vi "Auton and Setpoints Selector.vi"() -> ()   [LabVIEW 2014]
uses:
  <vilib>/Rock Robotics/WPI/Joystick/WPI_JoystickGetSetRefNum.vi
  Robot Global Data.vi
  <vilib>/Rock Robotics/Network Tables/SD Write String.vi
  <vilib>/Rock Robotics/Network Tables/SD Write Number.vi
panel:
  out "Setpoints File Selected 2":string
  out "Auton File Selected":string
  out "Number of Auton Files":i64
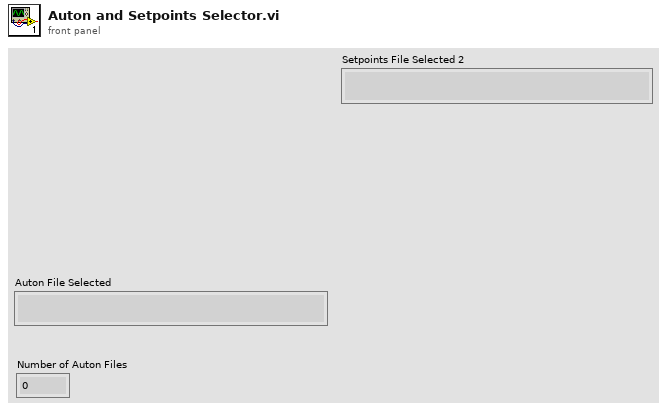
[diagram p1: front panel]
types:
  T1 = typedef "WPI_JoystickDevRef.ctl" = cluster{"Device":T2}
  T2 = typedef "WPI_JoystickDeviceEnum.ctl" = enum16{"USB 0", "USB 1", "USB 2", "USB 3", "USB 4", "USB 5"}
  T3 = cluster{"Buttons[0]":bool, "Buttons[1]":bool, "Buttons[2]":bool, "Buttons[3]":bool, "Buttons[4]":bool, "Buttons[5]":bool, "Buttons[6]":bool, "Buttons[7]":bool, "Buttons[8]":bool}
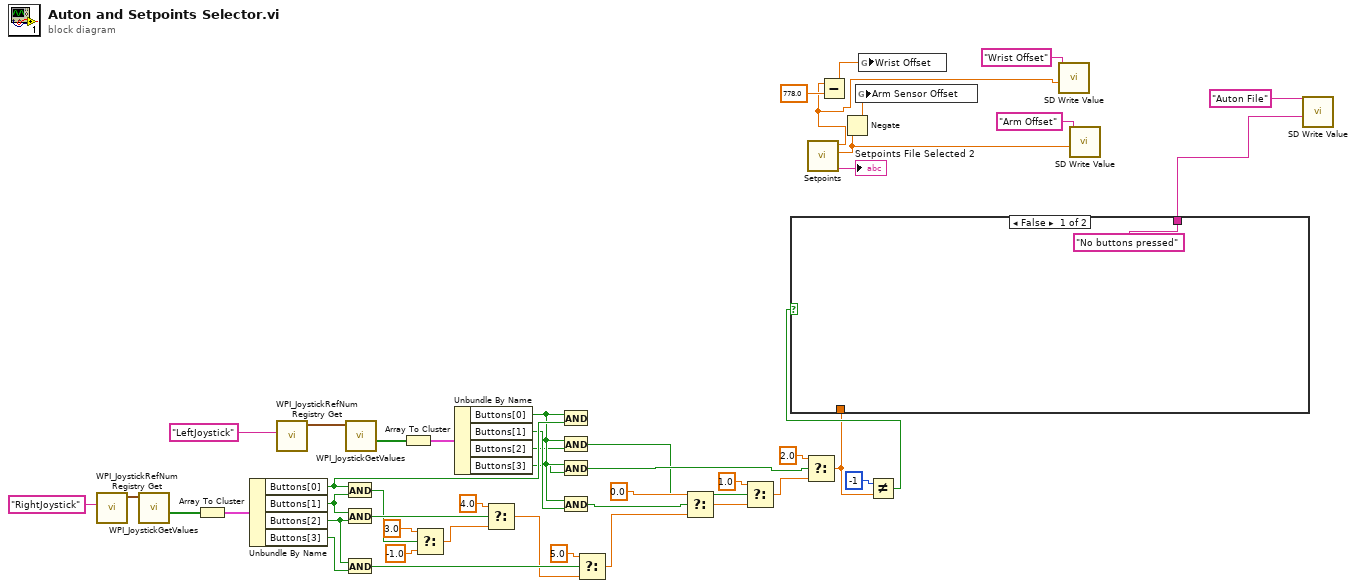
[diagram p0: block diagram]
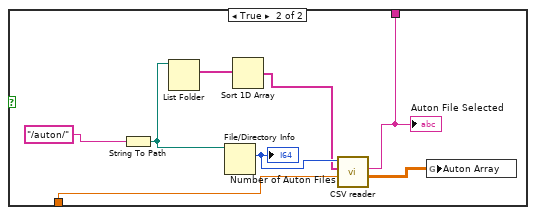
[diagram p2: hidden frame]
diagram:
  n1 = call <vilib>:"WPI_JoystickRefNum Registry Get.vi"("refnum name"="RightJoystick") -> ("JoystickDevRef"=w24:T1)  [unwired: 9 in, 1 out]
  n2 = call <vilib>:"WPI_JoystickGetValues.vi"("JoystickDevRef"=w24) -> ("Buttons"=w23:bool[])  [unwired: 6 in, 4 out]
  n3 = Array To Cluster(array=w23) -> (cluster=w22:T3)
  n4 = Unbundle By Name(w22) -> ("Buttons[0]"=w21:bool, "Buttons[1]"=w20:bool, "Buttons[2]"=w19:bool, "Buttons[3]"=w18:bool)
  n5 = call <vilib>:"WPI_JoystickRefNum Registry Get.vi"("refnum name"="LeftJoystick") -> ("JoystickDevRef"=w27:T1)  [unwired: 9 in, 1 out]
  n6 = And(x=w21, y=w20) -> (x .and. y?=w30:bool)
  n7 = And(x=w20, y=w19) -> (x .and. y?=w33:bool)
  n8 = And(x=w19, y=w18) -> (x .and. y?=w38:bool)
  n9 = call <vilib>:"WPI_JoystickGetValues.vi"("JoystickDevRef"=w27) -> ("Buttons"=w25:bool[])  [unwired: 6 in, 4 out]
  n10 = Array To Cluster(array=w25) -> (cluster=w17:T3)
  n11 = Select(t=3.0, s=w30, f=-1.0) -> (s? t:f=w34:dbl)
  n12 = Unbundle By Name(w17) -> ("Buttons[0]"=w16:bool, "Buttons[1]"=w15:bool, "Buttons[2]"=w14:bool, "Buttons[3]"=w13:bool)
  n13 = Select(t=4.0, s=w33, f=w34) -> (s? t:f=w36:dbl)
  n14 = And(x=w16, y=w21) -> ()  [unwired: 1 out]
  n15 = And(x=w16, y=w14) -> (x .and. y?=w43:bool)
  n16 = And(x=w16, y=w13) -> (x .and. y?=w46:bool)
  n17 = And(x=w16, y=w15) -> (x .and. y?=w45:bool)
  n18 = Select(t=5.0, s=w38, f=w36) -> (s? t:f=w47:dbl)
  n19 = Select(t=0.0, s=w45, f=w47) -> (s? t:f=w42:dbl)
  n20 = Select(t=1.0, s=w43, f=w42) -> (s? t:f=w40:dbl)
  n21 = Select(t=2.0, s=w46, f=w40) -> (s? t:f=w11:dbl)
  n22 = call "Setpoints.vi"() -> ("Setpoints File Selected"=→"Setpoints File Selected 2":string, "arm position offset"=w3:dbl, "wrist position offset"=w6:dbl)  [unwired: 7 in]
  n23 = Subtract(x=w6, y=778.0) -> (x-y=w9:dbl)
  n24 = Negate(x=w3) -> (-x=w7:dbl)
  n25 = global write "Robot Global Data.vi" "Arm Sensor Offset"(w7) -> ()
  n26 = global write "Robot Global Data.vi" "Wrist Offset"(w9) -> ()
  n27 = Not Equal?(x=-1, y=w11) -> (x != y?=w12:bool)
  n28 = case shown="False" w12 {
    tunnel: w11 -> [_ w51]
    tunnel: ["No buttons pressed" ("Auton File Selected") w49] -> w1
    frame False {
    }
    frame True {
      n29 = String To Path(string="/auton/") -> (path=w55:path)
      n30 = List Folder(path=w55) -> (filenames=w54:string[])  [unwired: 3 in, 3 out]
      n31 = File/Directory Info(path=w55) -> (size=w53:i64)  [unwired: 1 in, 6 out]
      "Number of Auton Files" <- w53
      n32 = Sort 1D Array(array=w54) -> (sorted array=w52:string[])
      n33 = call "CSV reader.vi"("x"=w51, "Array"=w52, "Number CSV"=w53) -> ("Auton Array"=w50:dbl[][], "Auton File Selected"=w49:string)  [unwired: 7 in]
      "Auton File Selected" <- w49
      n34 = global write "Robot Global Data.vi" "Auton Array"(w50) -> ()
    }
  }
  n35 = call-poly <vilib>:"SD Write Value.vi"("Numeric"=w6, "Name"="Wrist Offset") -> ()  [unwired: 8 in, 2 out]
  n36 = call-poly <vilib>:"SD Write Value.vi"("Numeric"=w3, "Name"="Arm Offset") -> ()  [unwired: 8 in, 2 out]
  n37 = call-poly <vilib>:"SD Write Value.vi"("String"=w1, "Name"="Auton File") -> ()  [unwired: 8 in, 2 out]
